vi "Actor Core.vi"(8 "error in":errorcluster, 11 "Chat Window in":refnum<class "Chat Window.lvclass">) -> (0 "error out":errorcluster, 3 "Actor out":refnum<class "Actor.lvclass">)   [LabVIEW 2020, in "Chat Window.lvlib" / "Chat Window.lvclass"]
doc: "(<B>Filename</B>: Actor Framework.lvlib:Actor.lvclass:Actor Core.vi)\n\nReceives messages to the actor, reacts to them, and initiates any error handling that may shut the actor down.\n\nDescendant classes may override this VI to append parallel tasks for the actor to complete while it handles messages. Overrides use the Call Parent Method node."
uses:
  Chat Window.lvclass
  <vilib>/ActorFramework/Actor/Actor.lvclass
  <vilib>/ActorFramework/Stop Msg/Stop Msg.lvclass
  <vilib>/ni/Actors/Network Endpoint Actors/Network Endpoint/Network Endpoint/Network Endpoint.lvclass
  Chat Window Messages/Display Text Msg/Display Text Msg.lvclass
  C:/Program Files (x86)/National Instruments/LabVIEW 2021/vi.lib/ActorFramework/Actor/Actor.lvclass
  <vilib>/ni/Actors/Network Endpoint Actors/Notifying Nested Endpoint/Notifying Nested Endpoint.lvclass
  C:/Program Files (x86)/National Instruments/LabVIEW 2021/vi.lib/ni/Actors/Network Endpoint Actors/Network Endpoint/Network Endpoint/Network Endpoint.lvclass
panel:
  out "Connected":bool
  in  "Send":bool
  out "Text to display":string
  in  "Text to send":string
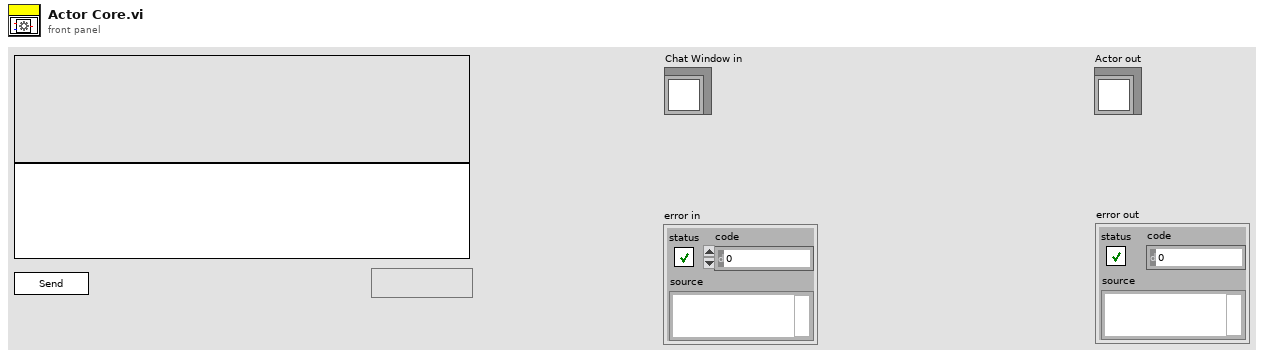
[diagram p1: front panel]
types:
  T1 = cluster{"Stop":refnum<user-event>, "Text":refnum<user-event>, "Connected":refnum<user-event>}
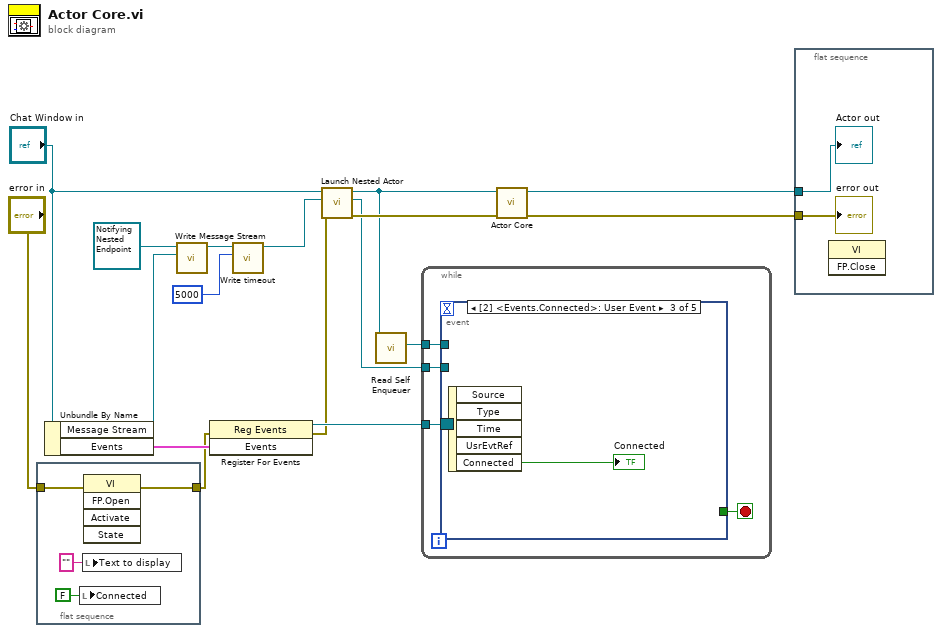
[diagram p0: block diagram]
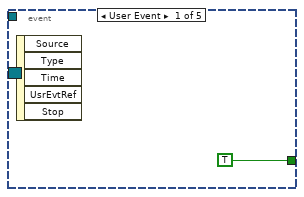
[diagram p2: hidden frame]
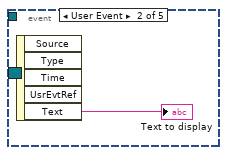
[diagram p3: hidden frame]
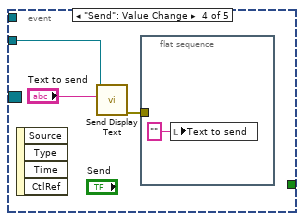
[diagram p4: hidden frame]
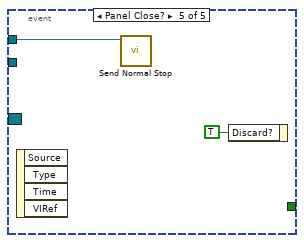
[diagram p5: hidden frame]
diagram:
  n1 = flat-sequence {
    tunnel: [w21] -> w8
    tunnel: "error in" -> [w18]
    frame #0 {
      n2 = local write "Connected"(FALSE ("Connected")) -> ()
      n3 = local write "Text to display"("" ("Text to display")) -> ()
      n4 = invoke class="VI" method="FP.Open"(error in=w18) -> (error out=w21:errorcluster)  [unwired: 4 in, 4 out]
    }
  }
  n5 = Unbundle By Name("Chat Window in") -> ("Message Stream"=w9:refnum<class "Message Stream.lvclass">, "Events"=w15:T1)
  n6 = call <vilib>:"Write Message Stream.vi"("Message Stream"=w9, "Network Endpoint in"=refnum<class "Notifying Nested Endpoint.lvclass"> refnum ("Notifying Nested Endpoint.lvclass")) -> ("Network Endpoint out"=w5:refnum<class "Notifying Nested Endpoint.lvclass">)  [unwired: 9 in]
  n7 = register-events(error in=w8, w15) -> (reference out=w14:refnum<event-registration>, error out=w1:errorcluster)  [unwired: 1 in]
  n8 = call <vilib>:"Write timeout.vi"("timeout"=5000, "Network Endpoint in"=w5) -> ("Network Endpoint out"=w3:refnum<class "Notifying Nested Endpoint.lvclass">)  [unwired: 9 in]
  n9 = call <vilib>:"Launch Nested Actor.vi"("error in (no error)"=w1, "Nested Actor"=w3, "Caller Actor in"="Chat Window in") -> ("error out"=w13:errorcluster, "Nested Actor's Enqueuer"=w12:refnum<class "Message Enqueuer.lvclass">, "Caller Actor out"=w6:refnum<class "Chat Window.lvclass">)  [unwired: 6 in]
  n10 = call <vilib>:"Read Self Enqueuer.vi"("Actor"=w6) -> ("Self Enqueuer"=w7:refnum<class "Message Enqueuer.lvclass">)  [unwired: 10 in]
  n11 = while {
    tunnel: w14 -> [w25]
    tunnel: w12 -> [w23]
    tunnel: w7 -> [w22]
    stop <- w24 stop-if-true
    n12 = event shown="[2] <Events.Connected>: User Event" {
      selector: w25 -> [_ _ _ _ _]
      dyn-events: _ -> [_ _ _ _ _]
      timeout: _ -> [_ _ _ _ _]
      tunnel: [TRUE _ _ _ _] -> w24
      tunnel: w23 -> [_ _ _ w31 _]
      tunnel: w22 -> [_ _ _ _ w33]
      event User Event {
        n13 = event-data() -> ()  [unwired: 1 in, 5 out]
      }
      event User Event {
        n14 = event-data() -> ("Text"=→"Text to display":string)  [unwired: 1 in, 4 out]
      }
      event User Event {
        n15 = event-data() -> ("Connected"=→"Connected":bool)  [unwired: 1 in, 4 out]
      }
      event "Send": Value Change {
        n16 = event-data() -> ()  [unwired: 1 in, 4 out]
        n17 = call "Send Display Text.vi"("Text"="Text to send", "Message Enqueuer"=w31) -> ("error out"=w29:errorcluster)  [unwired: 8 in, 1 out]
        n18 = flat-sequence {
          tunnel: w29 -> [_]
          frame #0 {
            n19 = local write "Text to send"("" ("Text to send")) -> ()
          }
        }
      }
      event Panel Close? {
        n20 = event-data() -> ()  [unwired: 1 in, 4 out]
        n21 = call <vilib>:"Send Normal Stop.vi"("Message Enqueuer"=w33) -> ()  [unwired: 10 in, 1 out]
        n22 = event-data("Discard?"=TRUE) -> ()  [unwired: 1 in, 1 out]
      }
    }
  }
  n23 = call-parent "Actor Core.vi"("error in"=w13, "Actor in"=w6) -> ("error out"=w17:errorcluster, "Actor out"=w16:refnum<class "Actor.lvclass">)  [unwired: 8 in]
  n24 = flat-sequence {
    tunnel: w17 -> [w36]
    tunnel: w16 -> [w35]
    frame #0 {
      n25 = invoke class="VI" method="FP.Close"() -> ()  [unwired: 3 in, 3 out]
      "error out" <- w36
      "Actor out" <- w35
    }
  }
